vi "DeviceInFIFO Read.vi"(8 "error in (no error)":errorcluster, 11 "DCM-NIVS-RT in":refnum<class "DCM-NIVS-RT.lvclass">) -> (0 "error out":errorcluster, 2 "DeviceInFIFO":refnum<k33>, 3 "DCM-NIVS-RT out":refnum<class "DCM-NIVS-RT.lvclass">)   [LabVIEW 2016, in "DCM Engine.lvlib" / "DCM-NIVS-RT.lvclass"]
uses:
  DCM-NIVS-RT.lvclass
  DCM-NIVS-RT.lvclass/DCM-NIVS-RT.ctl
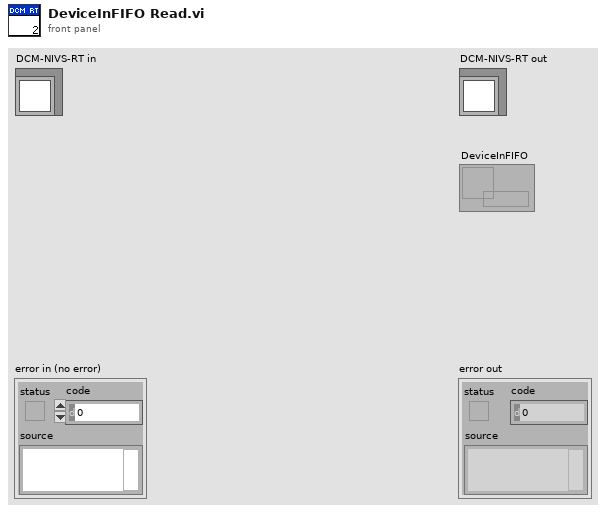
[diagram p1: front panel]
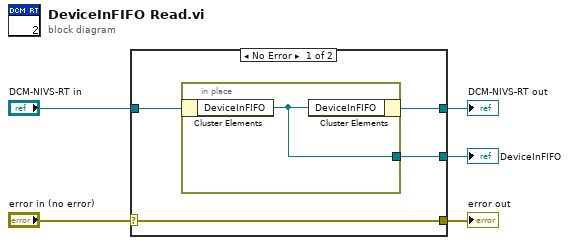
[diagram p0: block diagram]
diagram:
  n1 = case shown="No Error" "error in (no error)" {
    selector: "error in (no error)" -> [w9 w12]
    tunnel: [w9 w12] -> w4
    tunnel: [w6 w11] -> w2
    tunnel: "DCM-NIVS-RT in" -> [w8 w11]
    tunnel: [w7 _] -> w1
    frame No Error {
      n2 = in-place {
        in-place-border: [w10] -> w7
        n3 = in-place-cluster #1(w8) -> ("DeviceInFIFO"=w10:refnum<k33>)
        n4 = in-place-cluster #1("DeviceInFIFO"=w10) -> (w6:refnum<class "DCM-NIVS-RT.lvclass">)
      }
    }
    frame Error {
    }
  }
  "error out" <- w4
  "DCM-NIVS-RT out" <- w2
  "DeviceInFIFO" <- w1
